vi "search for alias.vi"(10 "alias":string, 11 "instance data":refnum<class "CEF_serializable configuration.lvclass">[](array[class])) -> (3 "index":i32)   [LabVIEW 2023, in "CEF.lvlib" / "CEF_serializable configuration.lvclass"]
doc: "Searches an object hierarchy for a given alias and returns the index of the first object which has this alias.Copyright 2017 National Instruments Corporation\n\nLicensed under the Apache License, Version 2.0 (the \"License\"); you may not use this file except in compliance with the License. You may obtain a copy of the License at http://www.apache.org/licenses/LICENSE-2.0\nUnless required by applicable law or agreed to in writing, software distributed under the License is distributed on an \"AS IS\" BASIS, WITHOUT WARRANTIES OR CONDITIONS OF ANY KIND, either express or implied. See the License for the specific language governing permissions and limitations under the License."
uses:
  serializable configuration/CEF_serializable configuration.lvclass
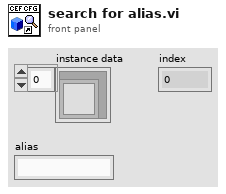
[diagram p1: front panel]
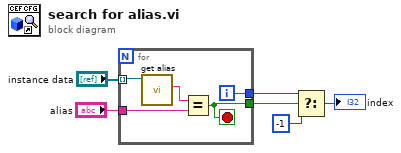
[diagram p0: block diagram]
diagram:
  n1 = for {
    tunnel: "instance data" -> [w8] mode=indexing
    tunnel: "alias" -> [w11]
    tunnel: [w10] -> w2
    tunnel: [w9] -> w4
    i -> [w10]
    stop <- w9 stop-if-true
    n2 = call "get alias.vi"("CEF_Configuration in"=w8) -> ("alias"=w7:string)  [unwired: 8 in, 2 out]
    n3 = Equal?(x=w7, y=w11) -> (x = y?=w9:bool)
  }
  n4 = Select(t=w2, s=w4, f=-1) -> (s? t:f=→"index":i32)
